vi "HeadDrawing.vi"(8 "error in (no error)":errorcluster, 11 "Snake in":refnum<class "Snake.lvclass">) -> (0 "error out":errorcluster, 3 "Snake out":refnum<class "Snake.lvclass">)   [LabVIEW 2014, in "Snake.lvclass"]
uses:
  Snake.lvclass
  Snake.lvclass/Snake.ctl
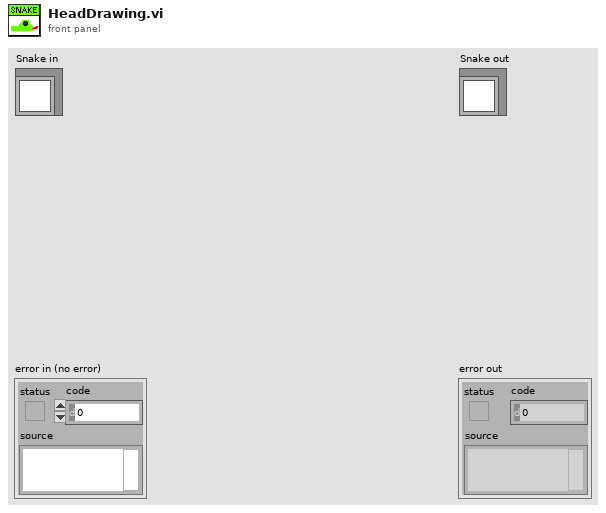
[diagram p1: front panel]
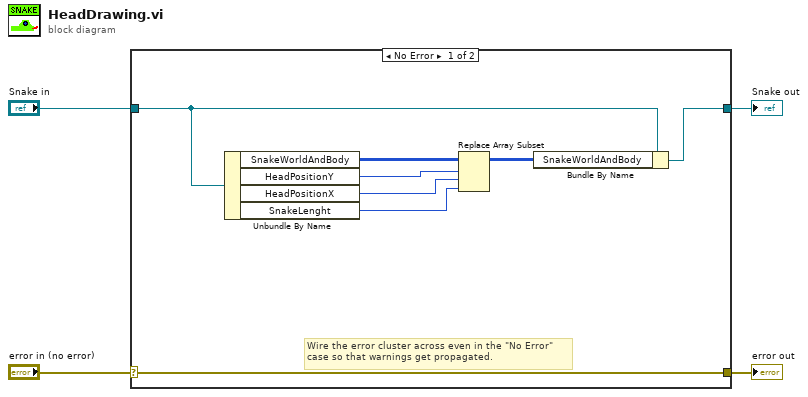
[diagram p0: block diagram]
diagram:
  n1 = case shown="No Error" "error in (no error)" {
    selector: "error in (no error)" -> [w12 w14]
    tunnel: [w12 w14] -> w3
    tunnel: [w6 w13] -> w1
    tunnel: "Snake in" -> [w11 w13]
    frame No Error {
      # "Wire the error cluster across even in the \"No Error\"\ncase so that warnings get propagated."
      n2 = Unbundle By Name(w11) -> ("SnakeWorldAndBody"=w10:u32[][], "HeadPositionY"=w9:i32, "HeadPositionX"=w8:i32, "SnakeLenght"=w7:u32)
      n3 = Replace Array Subset(array=w10, new element=w7, index (row)=w9, index (col)=w8) -> (w5:u32[][])
      n4 = Bundle By Name(cluster=w11, "SnakeWorldAndBody"=w5) -> (w6:refnum<class "Snake.lvclass">)
    }
    frame Error {
    }
  }
  "error out" <- w3
  "Snake out" <- w1
